vi "mcl_test.vi"() -> ()   [LabVIEW 2015, in "mcl_piezo.lvclass"]
uses:
  mcl_piezo.lvclass
panel:
  out "error out":errorcluster
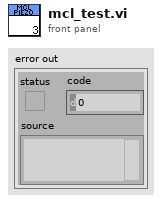
[diagram p1: front panel]
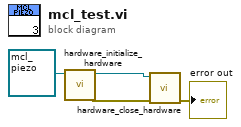
[diagram p0: block diagram]
diagram:
  n1 = call-dynamic "hardware_initialize_hardware.vi"("mcl_piezo in"=refnum<class "mcl_piezo.lvclass"> refnum) -> ("error out"=w3:errorcluster, "mcl_piezo out"=w4:refnum<class "mcl_piezo.lvclass">)  [unwired: 9 in]
  n2 = call-dynamic "hardware_close_hardware.vi"("error in (no error)"=w3, "mcl_piezo in"=w4) -> ("error out"=→"error out":errorcluster)  [unwired: 8 in, 1 out]
